vi "导出扫描测试数据.vi"(6 "导出数据选择":enum8{"False", "True", "Mixed"}(c332), 11 "数据":T1[](array[typedef])) -> (2 "突变电压":dbl[][](array[numeric]), 3 "扫描数据":dbl[][](array[numeric]))   [LabVIEW 2020]
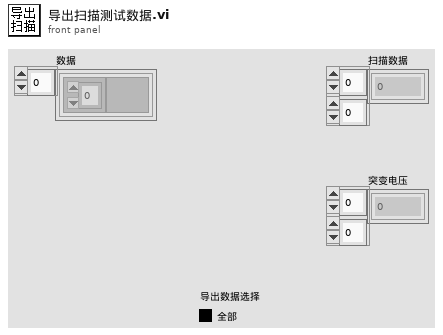
[diagram p1: front panel]
types:
  T1 = typedef "数据显示.xctl/波形数据定义.ctl" = cluster{"波形":dbl[][], "属性":variant}
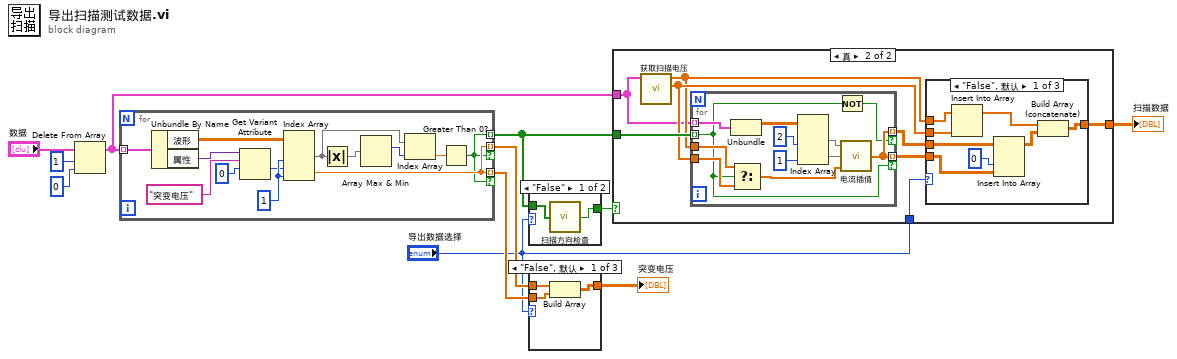
[diagram p0: block diagram]
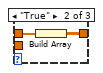
[diagram p2: hidden frame]
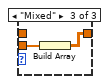
[diagram p3: hidden frame]
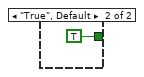
[diagram p4: hidden frame]
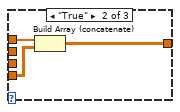
[diagram p6: hidden frame]
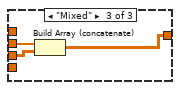
[diagram p7: hidden frame]
diagram:
  n1 = Delete From Array(array="数据", length=1 ("长度"), index=0 ("索引")) -> (array with subset deleted=w1:T1[])  [unwired: 1 out]
  n2 = for {
    tunnel: w1 -> [w24] mode=indexing
    tunnel: [w16] -> w8 mode=indexing if=w15
    tunnel: [w15] -> w11 mode=indexing
    tunnel: [w16] -> w7 mode=indexing if=w15
    w19 = 1 ("禁用的索引 (列)")
    n3 = Unbundle By Name(w24) -> ("波形"=w20:dbl[][], "属性"=w23:variant)
    n4 = Get Variant Attribute(Variant=w23, name="突变电压" ("名称"), default value (empty Variant)=0 ("突变电压")) -> (value=w18:i32)  [unwired: 1 in, 3 out]
    n5 = Index Array(array=w20, index (col) #1=w19, index (row) #2=w18, index (col) #2=w19) -> (element #1=w13:dbl[], element #2=w16:dbl)  [unwired: 1 in]
    n6 = Absolute Value(x=w13) -> (abs(x)=w14:dbl[])
    n7 = Array Max & Min(array=w14) -> (max index (indices)=w12:i32)  [unwired: 3 out]
    n8 = Index Array(array=w13, index=w12) -> (element=w17:dbl)
    n9 = Greater Than 0?(x=w17) -> (x > 0?=w15:bool)
  }
  n10 = case shown="\"False\"" "导出数据选择" {
    tunnel: w11 -> [w26 _]
    tunnel: [w25 TRUE ("检查通过？")] -> w9
    frame "False" {
      n11 = call "扫描方向检查.vi"("扫描方向"=w26) -> ("检查通过？"=w25:bool)
    }
    frame "True", Default {
    }
  }
  n12 = case shown="\"False\", 默认" "导出数据选择" {
    tunnel: w8 -> [w30 w32 _]
    tunnel: w7 -> [w29 _ w33]
    tunnel: [w28 w31 w34] -> w6
    frame "False", Default {
      n13 = Build Array(w30, w29) -> (w28:dbl[][])
    }
    frame "True" {
      n14 = Build Array(w32) -> (w31:dbl[][])
    }
    frame "Mixed" {
      n15 = Build Array(w33) -> (w34:dbl[][])
    }
  }
  "突变电压" <- w6
  n16 = case shown="真" w9 {
    tunnel: w11 -> [_ w42]
    tunnel: [_ w41] -> w10
    tunnel: "导出数据选择" -> [_ w40]
    tunnel: w1 -> [_ w35]
    frame False {
    }
    frame True {
      n17 = call "获取扫描电压.vi"("数据"=w35) -> ("负"=w37:dbl[], "正"=w36:dbl[])  [unwired: 9 in]
      n18 = for {
        tunnel: w35 -> [w68] mode=indexing
        tunnel: w42 -> [w60] mode=indexing
        tunnel: w36 -> [w63]
        tunnel: w37 -> [w62]
        tunnel: [w61] -> w39 mode=indexing if=w60
        tunnel: [w61] -> w38 mode=indexing if=w59
        n19 = Unbundle(w68) -> ("波形"=w67:dbl[][])  [unwired: 1 out]
        n20 = Select(t=w63, s=w60, f=w62) -> (s? t:f=w64:dbl[])
        n21 = Index Array(array=w67, index (col) #1=2 ("索引 (行)"), index (col) #2=1 ("索引 (行)")) -> (element #1=w66:dbl[], element #2=w65:dbl[])  [unwired: 2 in]
        n22 = Not(x=w60) -> (.not. x?=w59:bool)
        n23 = call "电流插值.vi"("电压"=w64, "原始电压"=w65, "原始电流"=w66) -> ("插值后电流"=w61:dbl[])
      }
      n24 = case shown="\"False\", 默认" w40 {
        tunnel: w36 -> [w50 w53 _]
        tunnel: w37 -> [w49 _ w55]
        tunnel: w39 -> [w48 w51 _]
        tunnel: w38 -> [w46 _ w54]
        tunnel: [w43 w52 w56] -> w41
        frame "False", Default {
          n25 = Insert Into Array(array=w50, new element=w49) -> (w45:dbl[])  [unwired: 1 in]
          n26 = Insert Into Array(array=w46, index (col)=0 ("索引 (列)"), new element=w48) -> (w44:dbl[][])  [unwired: 1 in]
          n27 = Build Array (concatenate)(w45, w44) -> (w43:dbl[][])
        }
        frame "True" {
          n28 = Build Array (concatenate)(w53, w51) -> (w52:dbl[][])
        }
        frame "Mixed" {
          n29 = Build Array (concatenate)(w55, w54) -> (w56:dbl[][])
        }
      }
    }
  }
  "扫描数据" <- w10
